vi "SendGlobalVariablesToNT.vi"(1 "Static Global Variable":refnum<vi>) -> ()   [LabVIEW 2019]
doc: "This VI sends all of the flagged data in a given global variable to the network table."
uses:
  1bf4823b-a618-4fa7-a86f-eba1a0a47ca9.vi
  dsdata.vi
  <vilib>/Rock Robotics/Network Tables/NT Write Boolean.vi
  <vilib>/Rock Robotics/Network Tables/NT Write Boolean Array.vi
  <vilib>/Rock Robotics/Network Tables/NT Write Number.vi
  <vilib>/Rock Robotics/Network Tables/NT Write Numeric Array.vi
  <vilib>/Rock Robotics/Network Tables/NT Write String.vi
  <vilib>/Rock Robotics/Network Tables/NT Write String Array.vi
  <vilib>/Utility/Data Type/NI_Data Type.lvlib
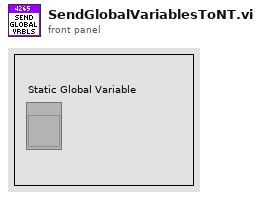
[diagram p1: front panel]
types:
  T1 = typedef "NI_Data Type.lvlib/Data Type.ctl" = enum8{"Invalid Type", "Void", "I8", "I16", "I32", "I64", "U8", "U16", "U32", "U64", "Single Float", "Double Float", "Extended Float", "Single Complex", "Double Complex", "Extended Complex", "Enum U8", "Enum U16", "Enum U32", "Enum U64", "Single Float With Unit", "Double Float With Unit", "Extended Float With Unit", "Single Complex with Unit", "Double Complex with Unit", "Extended Complex with Unit", "Boolean", "String", "Path", "Picture", "Tag", "Array", "Cluster", "Variant", "LV Variant", "Waveform", "Timestamp", "Digital Waveform", "Digital Data", "ExpressData", "Refnum", "External Data", "VI", "Poly VI", "LabVIEW Class Instance", "Fixed Point", "Set Collection", "Map Collection"}
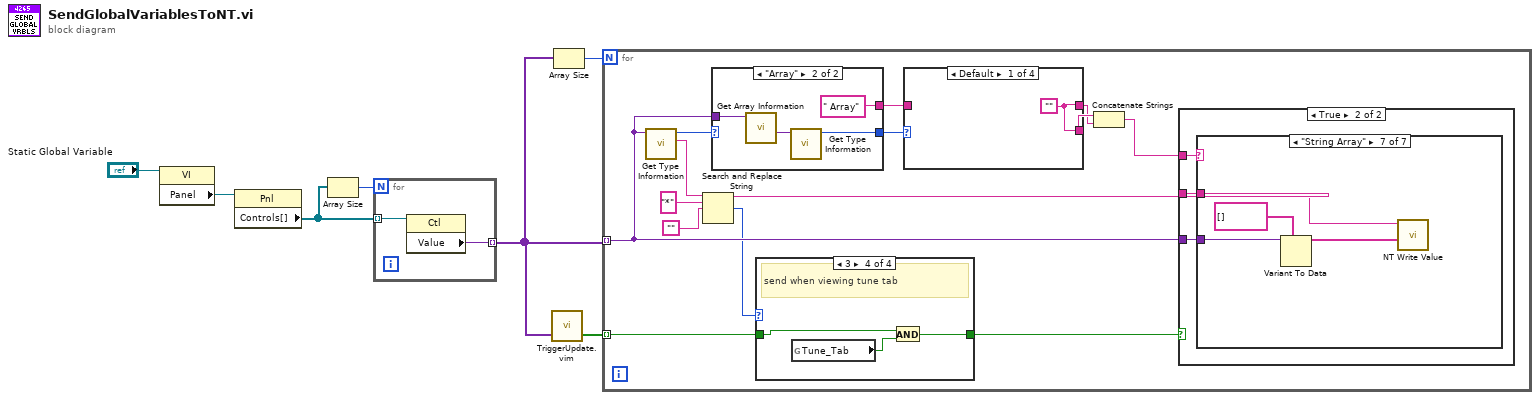
[diagram p0: block diagram]
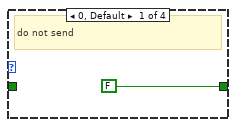
[diagram p2: hidden frame]
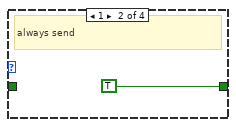
[diagram p3: hidden frame]
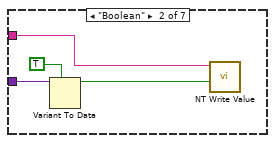
[diagram p7: hidden frame]
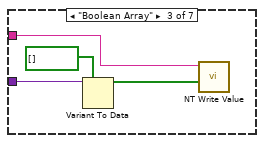
[diagram p8: hidden frame]
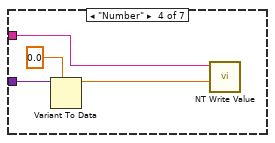
[diagram p9: hidden frame]
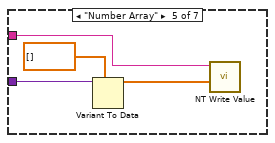
[diagram p10: hidden frame]
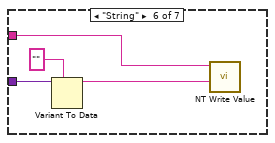
[diagram p11: hidden frame]
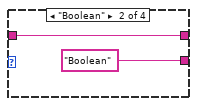
[diagram p12: hidden frame]
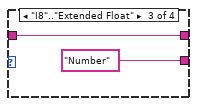
[diagram p13: hidden frame]
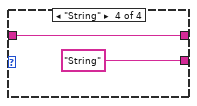
[diagram p14: hidden frame]
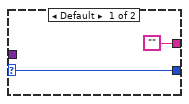
[diagram p15: hidden frame]
diagram:
  n1 = property class="VI"(reference="Static Global Variable") -> ("Panel"=w7:refnum<vi>)  [unwired: 1 in, 2 out]
  n2 = property class="Pnl"(reference=w7) -> ("Controls[]"=w4:refnum<vi>[])  [unwired: 1 in, 2 out]
  n3 = Array Size(array=w4) -> (size(s)=w3:i32)
  n4 = for {
    N: w3 -> [_]
    tunnel: w4 -> [w9] mode=indexing
    tunnel: [w8] -> w6 mode=indexing
    n5 = property class="Ctl"(reference=w9) -> ("Value"=w8:variant)  [unwired: 1 in, 2 out]
  }
  n6 = call "TriggerUpdate.vim"("Trigger"=w6) -> ("Update"=w2:bool[])  [unwired: 2 in]
  n7 = Array Size(array=w6) -> (size(s)=w5:i32)
  n8 = for {
    N: w5 -> [_]
    tunnel: w6 -> [w19] mode=indexing
    tunnel: w2 -> [w10] mode=indexing
    n9 = call <vilib>:"Get Type Information.vi"("variant"=w19) -> ("name"=w20:string, "type"=w18:T1)  [unwired: 6 in, 3 out]
    n10 = Search and Replace String(input string=w20, search string="*", replace string="") -> (result string=w21:string, number of replacements=w12:i32)  [unwired: 5 in, 2 out]
    n11 = case shown="\"Array\"" w18 {
      selector: w18 -> [w65 _]
      tunnel: w19 -> [_ w69]
      tunnel: [w65 w67] -> w17
      tunnel: ["" " Array"] -> w16
      frame Default {
      }
      frame "Array" {
        n12 = call <vilib>:"Get Array Information.vi"("variant"=w69) -> ("array element data type"=w68:variant)  [unwired: 7 in, 3 out]
        n13 = call <vilib>:"Get Type Information.vi"("variant"=w68) -> ("type"=w67:T1)  [unwired: 6 in, 4 out]
      }
    }
    n14 = case shown="3" w12 {
      tunnel: [FALSE TRUE w26 w28] -> w11
      tunnel: w10 -> [_ _ w26 w29]
      frame 0, Default {
        # "do not send"
      }
      frame 1 {
        # "always send"
      }
      frame 2 {
        # "send on change"
      }
      frame 3 {
        # "send when viewing tune tab"
        n15 = global read "dsdata.vi" "Tune_Tab"() -> (w27:bool)
        n16 = And(x=w29, y=w27) -> (x .and. y?=w28:bool)
      }
    }
    n17 = case shown="Default" w17 {
      tunnel: w16 -> [_ w59 w61 w63]
      tunnel: [w57 w59 w61 w63] -> w14
      tunnel: [w57 "Boolean" "Number" "String"] -> w15
      frame Default {
        w57 = ""
      }
      frame "Boolean" {
      }
      frame "I8".."Extended Float" {
      }
      frame "String" {
      }
    }
    n18 = Concatenate Strings(w15, w14) -> (w13:string)
    n19 = case shown="True" w11 {
      tunnel: w19 -> [_ w32]
      tunnel: w21 -> [_ w31]
      tunnel: w13 -> [_ w30]
      frame False {
      }
      frame True {
        n20 = case shown="\"String Array\"" w30 {
          tunnel: w32 -> [_ w35 w40 w44 w48 w52 w56]
          tunnel: w31 -> [_ w33 w38 w42 w46 w50 w54]
          frame Default {
          }
          frame "Boolean" {
            n21 = Variant To Data(type=TRUE, Variant=w35) -> (data=w34:bool)  [unwired: 1 in, 1 out]
            n22 = call-poly <vilib>:"NT Write Value.vi"("Boolean"=w34, "Name"=w33) -> ()  [unwired: 9 in, 1 out]
          }
          frame "Boolean Array" {
            n23 = Variant To Data(type=bool[] [], Variant=w40) -> (data=w39:bool[])  [unwired: 1 in, 1 out]
            n24 = call-poly <vilib>:"NT Write Value.vi"("Boolean Array"=w39, "Name"=w38) -> ()  [unwired: 9 in, 1 out]
          }
          frame "Number" {
            n25 = Variant To Data(type=0.0, Variant=w44) -> (data=w43:dbl)  [unwired: 1 in, 1 out]
            n26 = call-poly <vilib>:"NT Write Value.vi"("Numeric"=w43, "Name"=w42) -> ()  [unwired: 9 in, 1 out]
          }
          frame "Number Array" {
            n27 = Variant To Data(type=dbl[] [], Variant=w48) -> (data=w47:dbl[])  [unwired: 1 in, 1 out]
            n28 = call-poly <vilib>:"NT Write Value.vi"("Numeric Array"=w47, "Name"=w46) -> ()  [unwired: 9 in, 1 out]
          }
          frame "String" {
            n29 = Variant To Data(type="", Variant=w52) -> (data=w51:string)  [unwired: 1 in, 1 out]
            n30 = call-poly <vilib>:"NT Write Value.vi"("String"=w51, "Name"=w50) -> ()  [unwired: 9 in, 1 out]
          }
          frame "String Array" {
            n31 = Variant To Data(type=string[] [], Variant=w56) -> (data=w55:string[])  [unwired: 1 in, 1 out]
            n32 = call-poly <vilib>:"NT Write Value.vi"("String Array"=w55, "Name"=w54) -> ()  [unwired: 9 in, 1 out]
          }
        }
      }
    }
  }
